vi "Siargo Get Flow Rate.vi"(8 "error in (no error)":errorcluster, 11 "Modbus API in":refnum<class "Modbus API.lvclass">) -> (0 "error out":errorcluster, 2 "Flow Rate (SCFH)":dbl, 3 "Modbus API out":refnum<class "Modbus API.lvclass">)   [LabVIEW 2020]
uses:
  <vilib>/NI/Modbus Library/API/Modbus API.lvclass
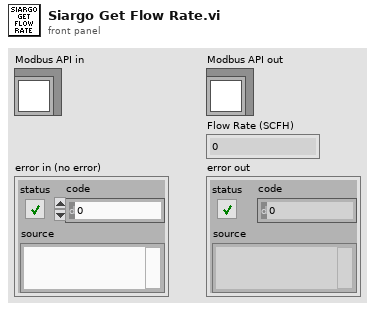
[diagram p1: front panel]
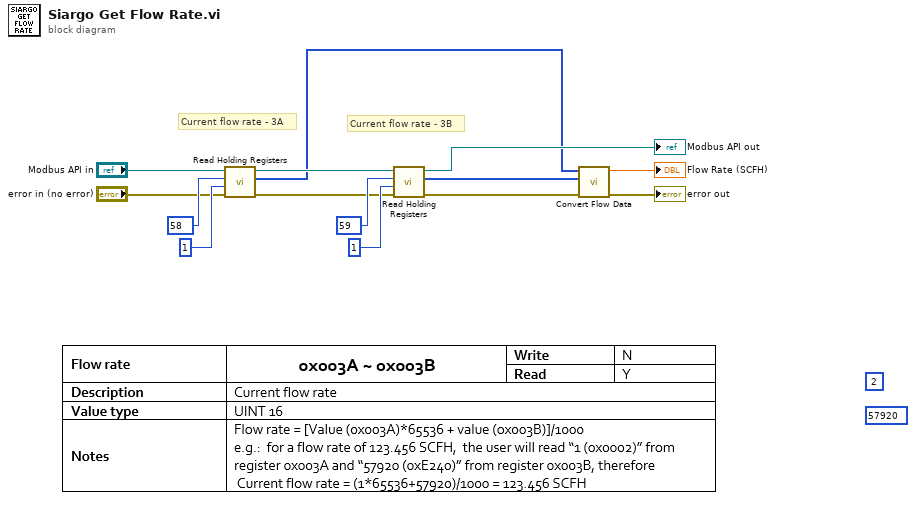
[diagram p0: block diagram]
diagram:
  (unwired) 57920
  (unwired) 2
  # "Current flow rate - 3B"
  # "Current flow rate - 3A"
  n1 = call-dynamic "Read Holding Registers.vi"("error in"="error in (no error)", "number of inputs"=u16 1, "starting address"=u16 58, "Modbus instance in"="Modbus API in") -> ("error out"=w8:errorcluster, "register values"=w5:u16[], "Modbus instance out"=w7:refnum<class "Modbus API.lvclass">)  [unwired: 5 in]
  n2 = call-dynamic "Read Holding Registers.vi"("error in"=w8, "number of inputs"=u16 1, "starting address"=u16 59, "Modbus instance in"=w7) -> ("error out"=w3:errorcluster, "register values"=w4:u16[], "Modbus instance out"=→"Modbus API out":refnum<class "Modbus API.lvclass">)  [unwired: 5 in]
  n3 = call "Convert Flow Data.vi"("error in (no error)"=w3, "register values - 3B"=w4, "register values - 3A"=w5) -> ("error out"=→"error out":errorcluster, "Flow Rate (SCFH)"=→"Flow Rate (SCFH)":dbl)  [unwired: 7 in]
